vi "RampVoltagewithDDSv5.vi"() -> ()   [LabVIEW 2016]
uses:
  <vilib>/DAQmx/write.llb/DAQmx Write (Analog 2D DBL NChan NSamp).vi
  <vilib>/DAQmx/create/channels.llb/DAQmx Create Channel (AO-Voltage-Basic).vi
  <vilib>/DAQmx/configure/timing.llb/DAQmx Timing (Sample Clock).vi
  <vilib>/DAQmx/configure/trigger.llb/DAQmx Start Trigger (Digital Edge).vi
  <vilib>/DAQmx/miscellaneous.llb/DAQmx Fill In Error Info.vi
  <resource>/objmgr/daqmx.rc
panel:
  in  "DDS delay [ms]":dbl
  in  "Plateau time (ms)":dbl=30.0
  out "Step seperation (us)":dbl=1.0
  in  "Ramp duration (us)":dbl=2000.0 format="%#_6f"
  in  "Ramp trigger source":T1(ring)=enum."BNC_IN_A_RISING"
  in  "Step Size (Hz)":dbl=50000.0 format="%#_6f"
  in  "End Frequency (Hz)":dbl=290000000.0 format="%#_13g"
  in  "Starting Frequency (Hz)":dbl=190000000.0 format="%#_6f"
  in  "Channels":T2(ring)=enum."Both channels"
  out "return count":u32=240
  out "error out":errorcluster={"status"=TRUE, "code"=-1073807339, "source"="VISA Read in RampVoltagewithDDSv4.vi"}
  out "read buffer":string="dcp spi:CFR2=0x1000080\r\nflexdds> dcp spi:DRL=0x4A3D70A430A3D70A\r\nflexdds> dcp spi:DRSS=0x346DC000346DC\r\nflexdds> dcp spi:DRR=0xFA00FA\r\nflexdds> dcp spi:CFR2=0x80080\r\nflexdds> dcp wait::BNC_IN_A_RISING\r\nflexdds> dcp update:u+d\r\nflexdds> dcp wait:4000000h:\r\nflexdds> dcp update:-d\r\nflexdds> dcp wait:250000h:\r\nflexdds> dcp update:u\r\nflexdds> dcp start\r\n\u001b[34m[   7041038 N shell] L:FPGA:DCP[0]: flushing 13 insts (80 bytes); FIFO 5/4096 entries (1 msec)\u001b[0m\r\n\u001b[34m[   7041039 N shell] L:FPGA:DCP[1]: flushing 13 insts (80 bytes); FIFO 5/4096 entries (0 msec)\u001b[0m\r\n\u001b[32m[   7041039 V shell] L:FPGA:DCP[0]..."
  out "Final instruction string":string="dcp spi:CFR2=0x1000080\rdcp spi:DRL=0x4A3D70A430A3D70A\rdcp spi:DRSS=0x346DC000346DC\rdcp spi:DRR=0xFA00FA\rdcp spi:CFR2=0x80080\rdcp wait::BNC_IN_A_RISING\rdcp update:u+d\rdcp wait:4000000h:\rdcp update:-d\rdcp wait:250000h:\rdcp update:u\rdcp start\r"
  in  "physical channels 3":tag="Dev4/ao2"
  out "appended array":dbl[](array[numeric])
  in  "Sinewave amp (V)":dbl format="%#_6f"
  in  "Sinewave duration (ms)":dbl=0.3 format="%#_13g"
  out "size(s)":i32=16846
  in  "Trigger delay NI (ms)":dbl
  out "Sample rate":dbl=500000.0
  in  "source":tag="/Dev4/PFI0"
  in  "physical channels 2":tag="Dev4/ao1"
  in  "physical channels":tag="Dev4/ao0"
  in  "Plateau duration (ms)":dbl=29.689999999999998 step=0.01
  in  "Ramp duration (ms)":dbl=2.0 step=0.01
  in  "No of samples in ramp":dbl=1000.0
  in  "Ramp Amplitude (V)}":dbl=0.09200000000000007 step=0.001
  in  "error in":errorcluster
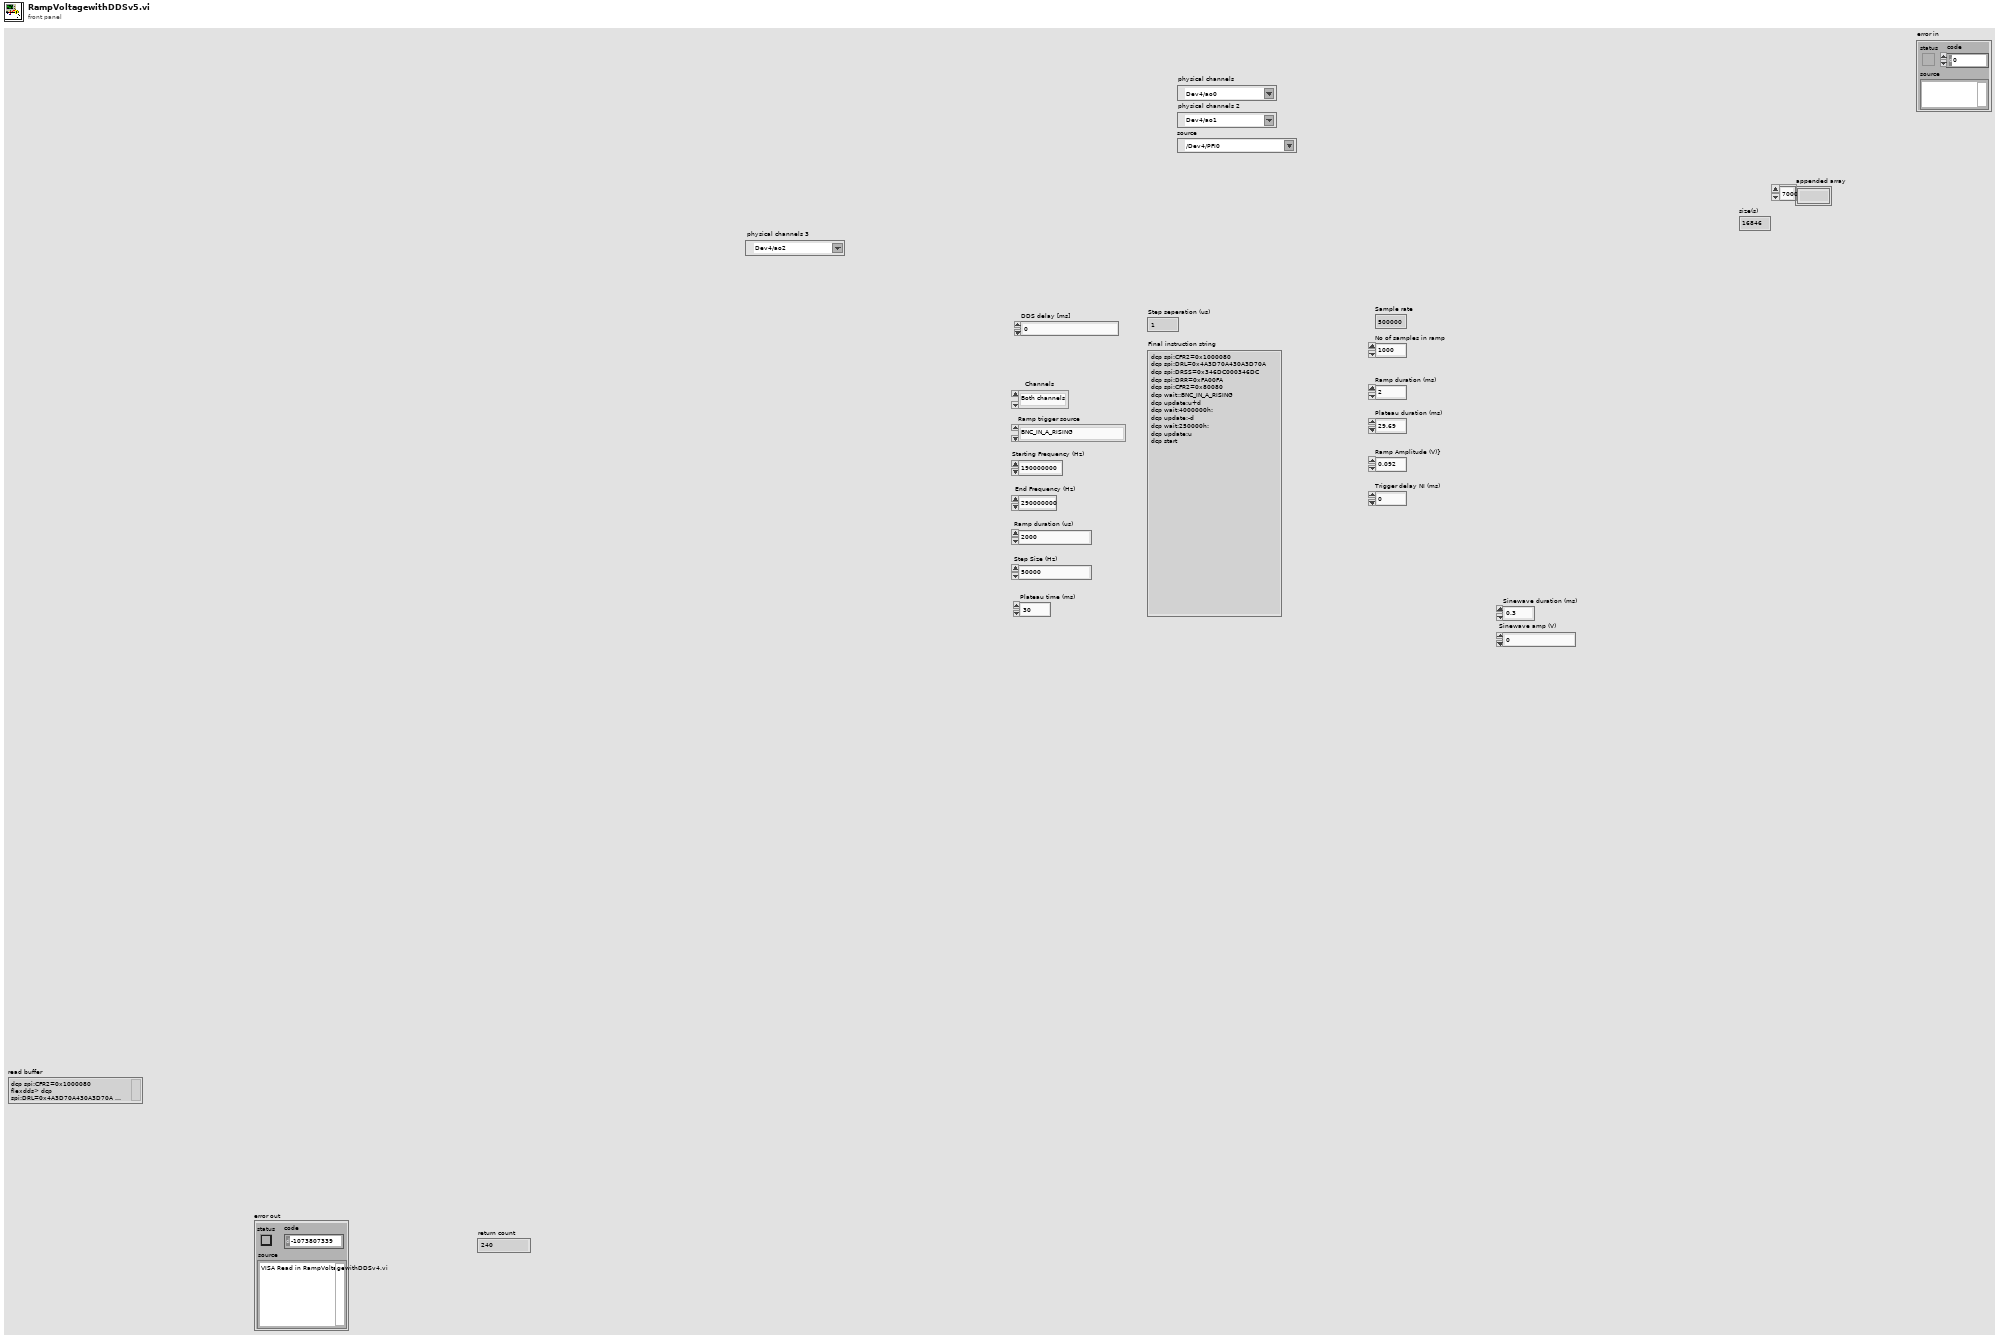
[diagram p1: front panel]
types:
  T1 = enum32{"O_RAMP_SWP_OVR", "RAM_SWP_OVR", "O_DROVER", "DROVER", "O_SPI_FIFO_EV1", "SPI_FIFO_EV1", "O_SPI_FIFO_EV0", "SPI_FIFO_EV0", "O_SPI_FIFO_FLUSHED", "SPI_FIFO_FLUSHED", "BNC_IN_B_LEVEL", "BNC_IN_B_FALLING", "BNC_IN_B_RISING", "BNC_IN_A_LEVEL", "BNC_IN_A_FALLING", "BNC_IN_A_RISING", "ALL_SPI_FIFOS_FLUSHED", "NONE"}
  T2 = enum32{"Channel 0", "Channel 1", "Both channels"}
  T3 = cluster{"Enable ASF from STP (F)":bool, "Digital ramp enable (F)":bool, "Digital ramp no-dwell high (F)":bool, "Digital ramp no-dwell low (F)":bool, "Matched latency enable (T)":bool, "Parallel data port enable (F)":bool}
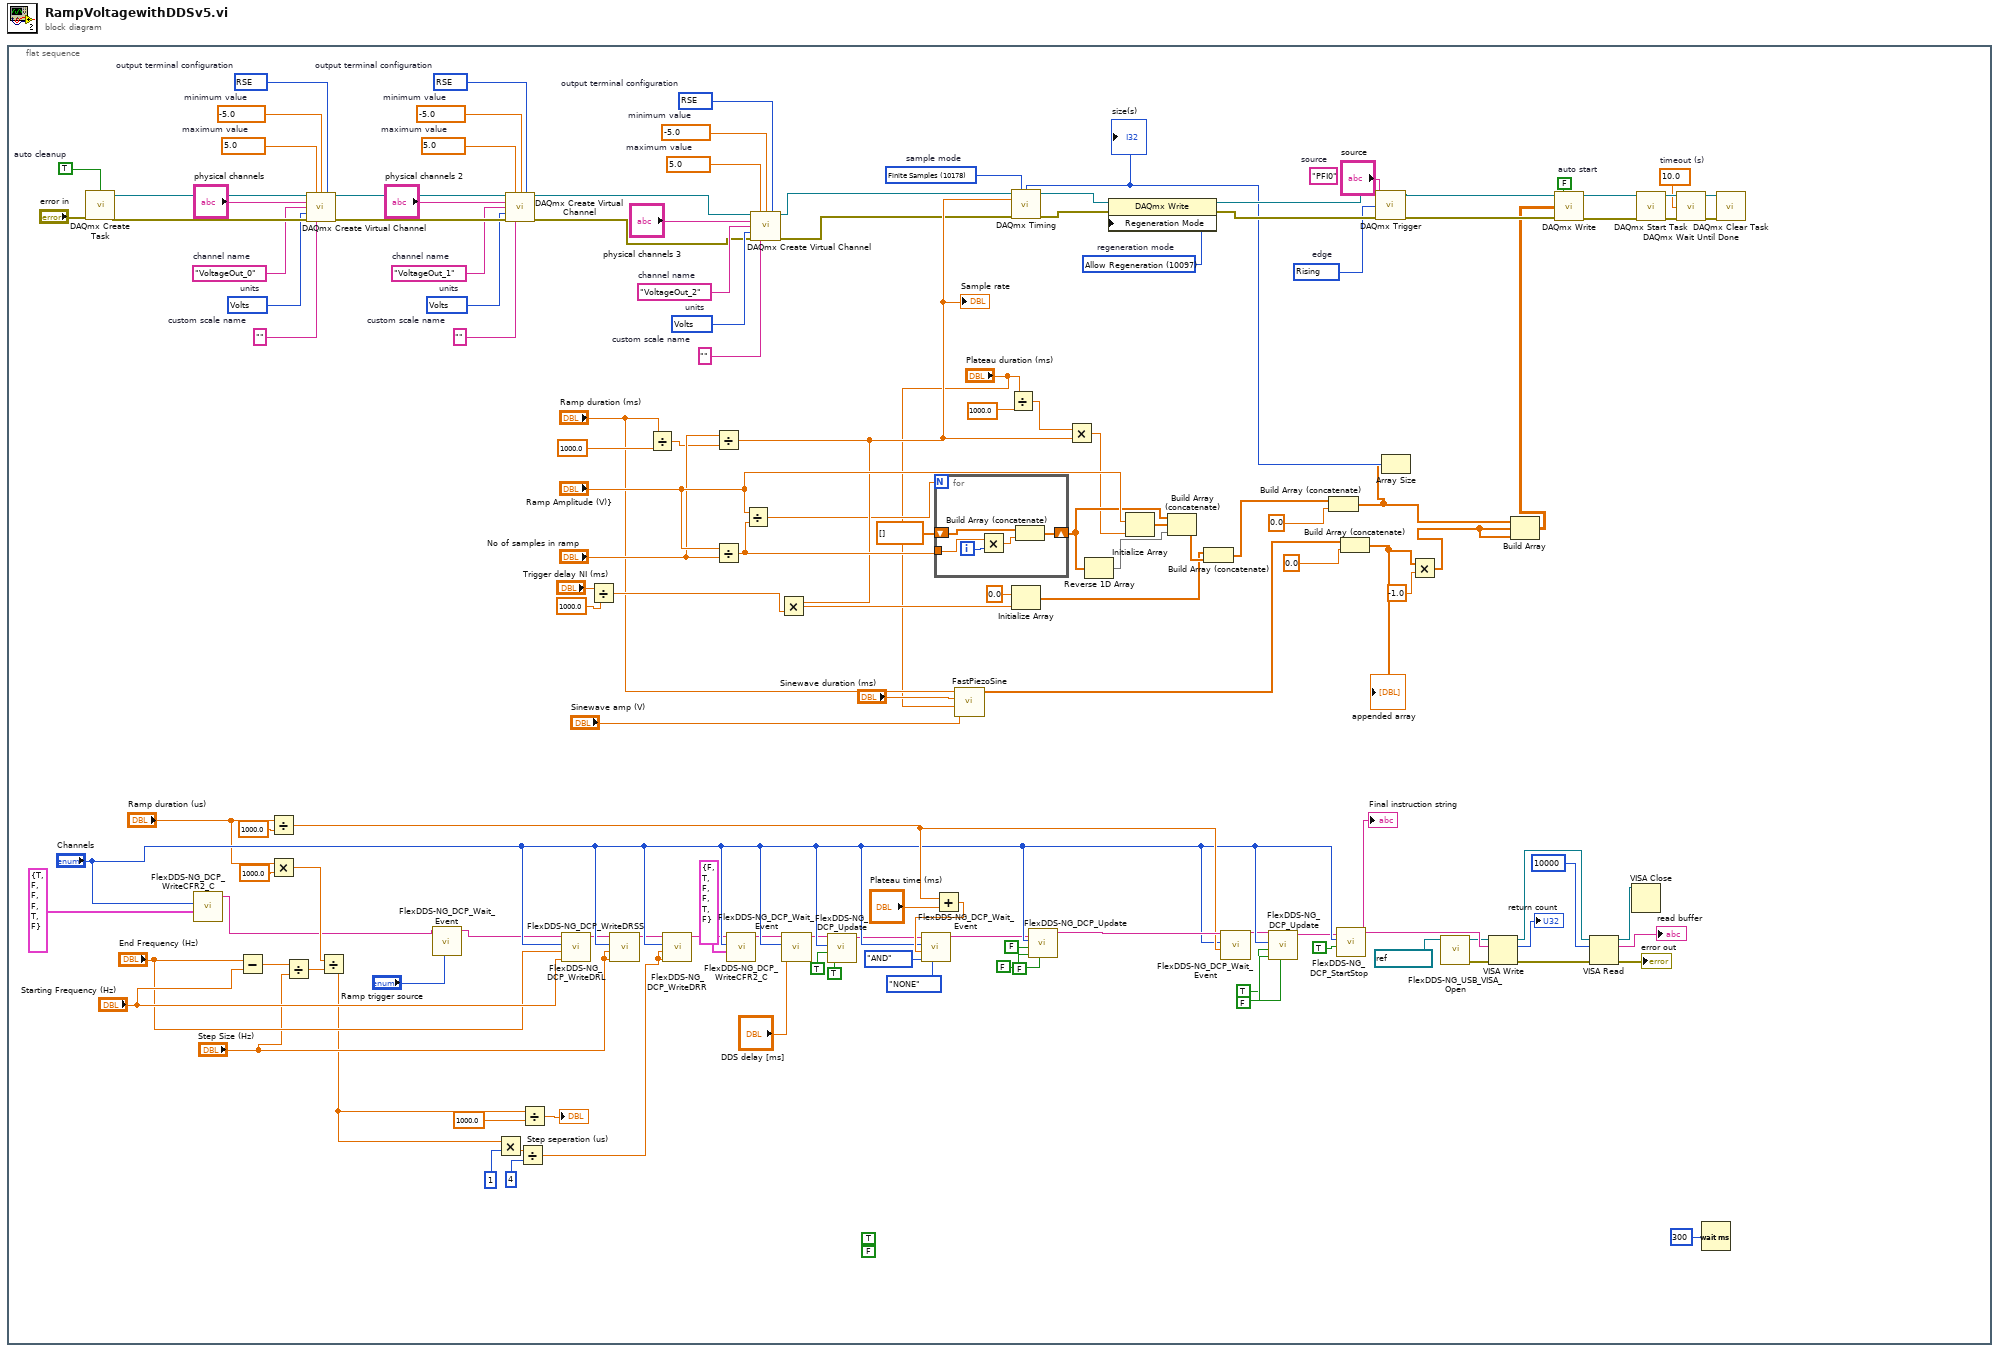
[diagram p0: block diagram]
diagram:
  n1 = flat-sequence {
    frame #0 {
      (unwired) TRUE ("Enable ASF from STP (F)")
      (unwired) FALSE ("Digital ramp enable (F)")
      w67 = 10083 items=["Default"=-1, "RSE"=10083, "Differential"=10106, "Pseudodifferential"=12529]  # output terminal configuration
      w68 = 10348 items=["Volts"=10348, "From Custom Scale"=10065]  # units
      w69 = "VoltageOut_2"  # channel name
      w70 = ""  # custom scale name
      w71 = -5.0  # minimum value
      w72 = 5.0  # maximum value
      w111 = 10280 items=["Rising"=10280, "Falling"=10171]  # edge
      (unwired) "PFI0"  # source
      w113 = 10097 items=["Allow Regeneration"=10097, "Do Not Allow Regeneration"=10158]  # regeneration mode
      w116 = 10178 items=["Finite Samples"=10178, "Continuous Samples"=10123, "Hardware Timed Single Point"=12522]  # sample mode
      w118 = 10083 items=["Default"=-1, "RSE"=10083, "Differential"=10106, "Pseudodifferential"=12529]  # output terminal configuration
      w119 = 10348 items=["Volts"=10348, "From Custom Scale"=10065]  # units
      w120 = "VoltageOut_1"  # channel name
      w121 = ""  # custom scale name
      w122 = -5.0  # minimum value
      w123 = 5.0  # maximum value
      w125 = 10083 items=["Default"=-1, "RSE"=10083, "Differential"=10106, "Pseudodifferential"=12529]  # output terminal configuration
      w126 = 10348 items=["Volts"=10348, "From Custom Scale"=10065]  # units
      w127 = "VoltageOut_0"  # channel name
      w129 = ""  # custom scale name
      w130 = -5.0  # minimum value
      w131 = 5.0  # maximum value
      w133 = TRUE  # auto cleanup
      w139 = 10.0  # timeout (s)
      w143 = FALSE  # auto start
      n2 = call <vilib>:"DAQmx Create Task.vi"("auto cleanup"=w133, "error in"="error in") -> ("task out"=w132:refnum<k21>, "error out"=w134:errorcluster)  [unwired: 12 in]
      n3 = call "FlexDDS-NG_DCP_WriteCFR2_C.vi"("CFR2 bits"=T3 {"Enable ASF from STP (F)"=TRUE, "Digital ramp enable (F)"=FALSE, "Digital ramp no-dwell high (F)"=FALSE, "Digital ramp no-dwell low (F)"=FALSE, "Matched latency enable (T)"=TRUE, "Parallel data port enable (F)"=FALSE} ("CFR2 bits 2"), "Channels"="Channels") -> ("appended instruction string"=w4:string)  [unwired: 9 in]
      n4 = Subtract(x="End Frequency (Hz)", y="Starting Frequency (Hz)") -> (x-y=w35:dbl)
      n5 = Divide(x="Ramp duration (us)", y=1000.0) -> (x/y=w55:dbl)
      n6 = Multiply(x="Ramp duration (us)", y=1000.0) -> (x*y=w38:dbl)
      n7 = Divide(x=w35, y="Step Size (Hz)") -> (x/y=w37:dbl)
      n8 = call-poly <vilib>:"DAQmx Create Virtual Channel.vi"("task in"=w132, "maximum value"=w131, "minimum value"=w130, "output terminal configuration"=w125, "physical channels"="physical channels", "name to assign"=w127, "units"=w126, "error in"=w134, "custom scale name"=w129) -> ("task out"=w124:refnum<k21>, "error out"=w128:errorcluster)  [unwired: 5 in]
      n9 = Divide(x=w38, y=w37) -> (x/y=w39:dbl)
      n10 = call "FlexDDS-NG_DCP_Wait_Event.vi"("Event 1"="Ramp trigger source", "appended instruction string in"=w4) -> ("appended instruction string"=w3:string)  [unwired: 9 in]
      n11 = Multiply(x=w39, y=u16 1) -> (x*y=w33:dbl)
      n12 = call-poly <vilib>:"DAQmx Create Virtual Channel.vi"("task in"=w124, "maximum value"=w123, "minimum value"=w122, "output terminal configuration"=w118, "physical channels"="physical channels 2", "name to assign"=w120, "units"=w119, "error in"=w128, "custom scale name"=w121) -> ("task out"=w65:refnum<k21>, "error out"=w64:errorcluster)  [unwired: 5 in]
      n13 = Divide(x=w33, y=u16 4) -> (x/y=w50:dbl)
      n14 = Divide(x=w39, y=1000.0 ("x/y")) -> (x/y=→"Step seperation (us)":dbl)
      n15 = call "FlexDDS-NG_DCP_WriteDRL.vi"("low limit"="Starting Frequency (Hz)", "high limit"="End Frequency (Hz)", "Channels"="Channels", "initial instruction string"=w3) -> ("appended instruction string"=w15:string)  [unwired: 7 in]
      n16 = Divide(x="Trigger delay NI (ms)", y=1000.0) -> (x/y=w87:dbl)
      n17 = call "FlexDDS-NG_DCP_WriteDRSS.vi"("increment step size"="Step Size (Hz)", "decrement step size"="Step Size (Hz)", "Channels"="Channels", "initial instruction string"=w15) -> ("appended instruction string"=w16:string)  [unwired: 7 in]
      n18 = Divide(x="Ramp duration (ms)", y=1000.0) -> (x/y=w102:dbl)
      n19 = call "FlexDDS-NG_DCP_WriteDRR.vi"("digital ramp positive slope rate"=w50, "digital ramp negative slope rate"=w50, "Channels"="Channels", "initial instruction string"=w16) -> ("appended instruction string"=w17:string)  [unwired: 7 in]
      n20 = Divide(x="No of samples in ramp", y=w102) -> (x/y=w86:dbl)
      "Sample rate" <- w86
      n21 = Divide(x="Ramp Amplitude (V)}", y="No of samples in ramp") -> (x/y=w109:dbl)
      n22 = call "FlexDDS-NG_DCP_WriteCFR2_C.vi"("CFR2 bits"=T3 {"Enable ASF from STP (F)"=FALSE, "Digital ramp enable (F)"=TRUE, "Digital ramp no-dwell high (F)"=FALSE, "Digital ramp no-dwell low (F)"=FALSE, "Matched latency enable (T)"=TRUE, "Parallel data port enable (F)"=FALSE}, "Channels"="Channels", "initial instruction string"=w17) -> ("appended instruction string"=w22:string)  [unwired: 8 in]
      n23 = Divide(x="Ramp Amplitude (V)}", y=w109) -> (x/y=w83:dbl)
      n24 = call-poly <vilib>:"DAQmx Create Virtual Channel.vi"("task in"=w65, "maximum value"=w72, "minimum value"=w71, "output terminal configuration"=w67, "physical channels"="physical channels 3", "name to assign"=w69, "units"=w68, "error in"=w64, "custom scale name"=w70) -> ("task out"=w63:refnum<k21>, "error out"=w62:errorcluster)  [unwired: 5 in]
      n25 = Multiply(x=w86, y=w87) -> (x*y=w85:dbl)
      n26 = call "FlexDDS-NG_DCP_Wait_Event.vi"("waiting time [ms]"="DDS delay [ms]", "Channels in"="Channels", "appended instruction string in"=w22) -> ("appended instruction string"=w23:string)  [unwired: 8 in]
      n27 = call "FlexDDS-NG_DCP_Update.vi"("DRCTL(true=+, false=-)"=TRUE, "IO_UPDATE(true=u, false = '')"=TRUE, "Channels"="Channels", "appended instruction string in"=w23) -> ("appended instruction string out"=w25:string)  [unwired: 7 in]
      n28 = for {
        N: w83 -> [_]
        shift-right: [w146] -> w107
        shift-left: dbl[] [] -> [w145]
        tunnel: w109 -> [w144]
        i -> [w148]
        n29 = Multiply(x=w144, y=w148) -> (x*y=w147:dbl)
        n30 = Build Array (concatenate)(w145, w147) -> (w146:dbl[])
      }
      n31 = Add(x=w55, y="Plateau time (ms)") -> (x+y=w57:dbl)
      n32 = call "FlexDDS-NG_DCP_Wait_Event.vi"("Event 1"=T1."NONE", "AND/OR"=enum32{"AND", "OR"}."AND", "waiting time [ms]"=w57, "Channels in"="Channels", "appended instruction string in"=w25) -> ("appended instruction string"=w52:string)  [unwired: 6 in]
      n33 = call "FastPiezoSine.vi"("Sinewave amp (V)"="Sinewave amp (V)", "Plateau duration (ms)"="Plateau duration (ms)", "Sinewave duration (ms)"="Sinewave duration (ms)", "Ramp duration (ms)"="Ramp duration (ms)") -> ("appended array"=w76:dbl[])  [unwired: 7 in]
      n34 = Divide(x="Plateau duration (ms)", y=1000.0) -> (x/y=w98:dbl)
      n35 = Initialize Array(0.0 ("element"), w85) -> (w90:dbl[])
      n36 = call "FlexDDS-NG_DCP_Update.vi"("ONLY IO_UPDATE"=FALSE, "DRCTL(true=+, false=-)"=FALSE ("DRCTL(true=+, false=-) 2"), "IO_UPDATE(true=u, false = '')"=FALSE ("IO_UPDATE(true=u, false = '')  2"), "Channels"="Channels", "appended instruction string in"=w52) -> ("appended instruction string out"=w58:string)  [unwired: 6 in]
      n37 = Multiply(x=w98, y=w86) -> (x*y=w97:dbl)
      n38 = Reverse 1D Array(array=w107) -> (reversed array=w105:dbl[])
      n39 = Initialize Array("Ramp Amplitude (V)}", w97) -> (w106:dbl[])
      n40 = Build Array (concatenate)(w107, w106, w105) -> (w91:dbl[])
      n41 = Build Array (concatenate)(w90, w91) -> (w79:dbl[])
      n42 = call "FlexDDS-NG_DCP_Wait_Event.vi"("waiting time [ms]"=w55, "Channels in"="Channels", "appended instruction string in"=w58) -> ("appended instruction string"=w31:string)  [unwired: 8 in]
      n43 = call "FlexDDS-NG_DCP_Update.vi"("ONLY IO_UPDATE"=TRUE, "DRCTL(true=+, false=-)"=FALSE ("DRCTL(true=+, false=-) 2"), "IO_UPDATE(true=u, false = '')"=TRUE ("IO_UPDATE(true=u, false = '')  2"), "Channels"="Channels", "appended instruction string in"=w31) -> ("appended instruction string out"=w29:string)  [unwired: 6 in]
      n44 = Build Array (concatenate)(w79, 0.0 ("y")) -> (w75:dbl[])
      n45 = call "FlexDDS-NG_DCP_StartStop.vi"("start (T) stop (F)"=TRUE, "Channels"="Channels", "initial instruction string"=w29) -> ("appended instruction string"=w45:string)  [unwired: 8 in]
      "Final instruction string" <- w45
      n46 = Build Array (concatenate)(w76, 0.0 ("y")) -> (w74:dbl[])
      "appended array" <- w74
      n47 = Array Size(array=w75) -> (size(s)=w96:i32)
      "size(s)" <- w96
      n48 = call-poly <vilib>:"DAQmx Timing.vi"("task/channels in"=w63, "sample mode"=w116, "samples per channel"=w96, "rate"=w86, "error in"=w62) -> ("task out"=w115:refnum<k21>, "error out"=w117:errorcluster)  [unwired: 9 in]
      n49 = property class="DAQmx Write"(reference=w115, error in=w117, "Regeneration Mode"=w113) -> (reference out=w112:refnum<k21>, error out=w114:errorcluster)
      n50 = call-poly <vilib>:"DAQmx Trigger.vi"("task/channels in"=w112, "source"="source", "edge"=w111, "error in"=w114) -> ("task out"=w101:refnum<k21>, "error out"=w100:errorcluster)  [unwired: 10 in]
      n51 = Multiply(x=w74, y=-1.0 ("element")) -> (x*y=w61:dbl[])
      n52 = call "FlexDDS-NG_USB_VISA_Open.vi"("FlexDDS-NG USB VISA resource name (COM)"=refnum<visa-resource-name> "COM7") -> ("error out"=w13:errorcluster, "FlexDDS-NG USB VISA resource name out"=w12:refnum<visa-resource-name>)  [unwired: 9 in]
      n53 = VISA Write(VISA resource name=w12, write buffer=w45, error in (no error)=w13) -> (VISA resource name out=w8:refnum<visa-resource-name>, return count=→"return count":u32, error out=w10:errorcluster)
      n54 = Build Array(w75, w61, w61) -> (w84:dbl[][])
      n55 = call-poly <vilib>:"DAQmx Write.vi"("task/channels in"=w101, "auto start"=w143, "data"=w84, "error in"=w100) -> ("task out"=w138:refnum<k21>, "error out"=w137:errorcluster)  [unwired: 9 in, 1 out]
      n56 = VISA Read(VISA resource name=w8, byte count=u32 10000, error in (no error)=w10) -> (VISA resource name out=w5:refnum<visa-resource-name>, read buffer=→"read buffer":string, error out=→"error out":errorcluster)  [unwired: 1 out]
      n57 = VISA Close(VISA resource name=w5) -> ()  [unwired: 1 in, 1 out]
      n58 = call <vilib>:"DAQmx Start Task.vi"("task/channels in"=w138, "error in"=w137) -> ("task out"=w142:refnum<k21>, "error out"=w141:errorcluster)  [unwired: 12 in]
      n59 = call <vilib>:"DAQmx Wait Until Done.vi"("task/channels in"=w142, "timeout (sec)"=w139, "error in"=w141) -> ("task out"=w136:refnum<k21>, "error out"=w140:errorcluster)  [unwired: 11 in]
      n60 = Wait (ms)(milliseconds to wait=u32 300) -> ()  [unwired: 1 out]
      n61 = call <vilib>:"DAQmx Clear Task.vi"("task in"=w136, "error in"=w140) -> ()  [unwired: 13 in, 1 out]
    }
  }
